vi "题目3温度测量子VI.vi"() -> ()   [LabVIEW 2017]
panel:
  out "字符串":string
  out "温度计":dbl(slide) scale=0.0..100.0
  in  "停止":bool
  in  "温度单位":bool
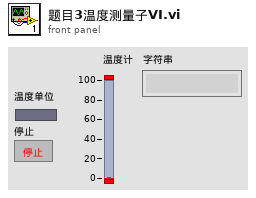
[diagram p1: front panel]
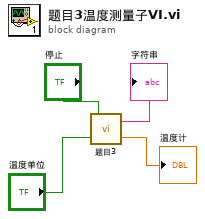
[diagram p0: block diagram]
diagram:
  n1 = call "题目3.vi"("温度单位"="温度单位", "停止"="停止") -> ("温度计"=→"温度计":dbl, "字符串"=→"字符串":string)
